vi "current version.vi"() -> ()   [LabVIEW 2015, in "SystemLink File configuration.lvclass"]
doc: "#CodeRequired\nThis global variable stores the current version of the module and should be updated as serialization formats change."
uses:
  SystemLink File configuration.lvclass
panel:
  out "current version":string="1.1.0.0"
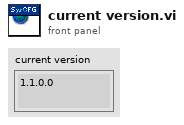
[diagram p1: front panel]
diagram:
